vi "Finish.vi"   [LabVIEW 2018]
doc: "This VI is called just before exiting. It is expected to close I/O refnum, save collected data, etc."
uses:
  <vilib>/Rock Robotics/WPI/Utilities/WPI_GetSetVariantRefNum.vi
types:
  T1 = typedef "WPI_JoystickDevRef.ctl" = cluster{"Device":T2}
  T2 = typedef "WPI_JoystickDeviceEnum.ctl" = enum16{"USB 0", "USB 1", "USB 2", "USB 3", "USB 4", "USB 5"}
  T3 = typedef "WPI_SolenoidDevRef.ctl" = cluster{"DevStatus":errorcluster, "Pneumatics Control Module":u8, "Forward Solenoid Channel":T4, "Reverse Solenoid Channel":T4}
  T4 = typedef "WPI_SolenoidChannel.ctl" = enum8{"Solenoid 0", "Solenoid 1", "Solenoid 2", "Solenoid 3", "Solenoid 4", "Solenoid 5", "Solenoid 6", "Solenoid 7", "Invalid"}
  T5 = typedef "WPI_CompressorDevRef.ctl" = cluster{"DevStatus":errorcluster, "Pneumatics Control Module":u8}
  T6 = typedef "WPI_SwitchDevRef.ctl" = cluster{"DevStatus":errorcluster, "DIO Channel":T7, "CntIndex":T8, "Normally Closed":bool}
  T7 = typedef "FPGA_DIOChannel.ctl" = enum8{"DIO 0", "DIO 1", "DIO 2", "DIO 3", "DIO 4", "DIO 5", "DIO 6", "DIO 7", "DIO 8", "DIO 9", "DIO MXP 0", "DIO MXP 1", "DIO MXP 2", "DIO MXP 3", "DIO MXP 4", "DIO MXP 5", "DIO MXP 6", "DIO MXP 7", "DIO MXP 8", "DIO MXP 9", "DIO MXP 10", "DIO MXP 11", "DIO MXP 12", "DIO MXP 13", "DIO MXP 14", "DIO MXP 15", "SPI Port CS1", "SPI Port CS2", "SPI Port CS3", "SPI Port MISO", "SPI Port MOSI", "Invalid"}
  T8 = typedef "FPGA_CounterCtrSystemIndex.ctl" = enum8{"Ctr 0", "Ctr 1", "Ctr 2", "Ctr 3", "Ctr 4", "Ctr 5", "Ctr 6", "Ctr 7", "Invalid"}
  T9 = typedef "WPI_MotorControlDeviceRef.ctl" = cluster{"DeviceStatus":errorcluster, "Type":T10, "PWM":cluster{"PWM Channel":T11, "DeadBand":T12}, "CAN":cluster{"Device Number":u8, "SetOutput VI Ref":variant, "GetOutput VI Ref":variant, "Enable VI Ref":variant, "Disable VI Ref":variant, "Data":variant}, "Invert":bool, "DIO PWM":cluster{"PWM \"Enable\" Channel":T11, "DIOChannel":T7, "PWM Rate":dbl}}
  T10 = typedef "WPI_MotorControlType.ctl" = enum16{"PWM", "CAN", "DIO PWM"}
  T11 = typedef "FPGA_DIOPWMChannel.ctl" = enum8{"PWM 0", "PWM 1", "PWM 2", "PWM 3", "PWM 4", "PWM 5", "PWM 6", "PWM 7", "PWM 8", "PWM 9", "PWM MXP 0", "PWM MXP 1", "PWM MXP 2", "PWM MXP 3", "PWM MXP 4", "PWM MXP 5", "PWM MXP 6", "PWM MXP 7", "PWM MXP 8", "PWM MXP 9", "Invalid"}
  T12 = typedef "WPI_PWMDeadband.ctl" = cluster{"Name":string, "maxPositivePwm":i32, "minPositivePwm":i32, "centerPwm":i32, "maxNegativePwm":i32, "minNegativePwm":i32, "angularRange":u16}
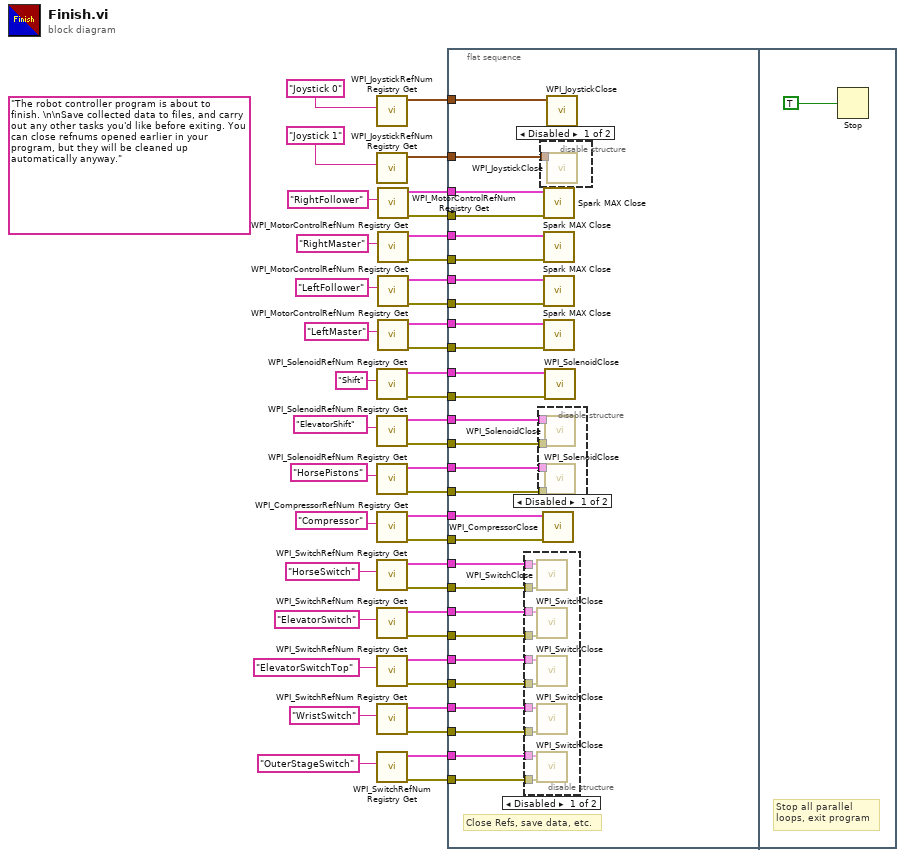
[diagram p0: block diagram]
diagram:
  (unwired) "The robot controller program is about to finish. \n\nSave collected data to files, and carry out any other tasks you'd like before exiting. You can close refnums opened earlier in your program, but they will be cleaned up automatically anyway."
  n1 = call <vilib>:"WPI_JoystickRefNum Registry Get.vi"("refnum name"="Joystick 0") -> ("JoystickDevRef"=w42:T1)  [unwired: 1 in, 9 out]
  n2 = call <vilib>:"WPI_JoystickRefNum Registry Get.vi"("refnum name"="Joystick 1") -> ("JoystickDevRef"=w17:T1)  [unwired: 1 in, 9 out]
  n3 = call <vilib>:"WPI_SolenoidRefNum Registry Get.vi"("refnum name"="Shift") -> ("error out"=w28:errorcluster, "SolenoidDevRef"=w29:T3)  [unwired: 9 in]
  n4 = call <vilib>:"WPI_SolenoidRefNum Registry Get.vi"("refnum name"="ElevatorShift") -> ("error out"=w22:errorcluster, "SolenoidDevRef"=w21:T3)  [unwired: 9 in]
  n5 = call <vilib>:"WPI_SolenoidRefNum Registry Get.vi"("refnum name"="HorsePistons") -> ("error out"=w25:errorcluster, "SolenoidDevRef"=w26:T3)  [unwired: 9 in]
  n6 = call <vilib>:"WPI_CompressorRefNum Registry Get.vi"("refnum name"="Compressor") -> ("error out"=w19:errorcluster, "CompressorDevRef"=w20:T5)  [unwired: 9 in]
  n7 = call <vilib>:"WPI_SwitchRefNum Registry Get.vi"("refnum name"="HorseSwitch") -> ("error out"=w13:errorcluster, "SwitchDevRef"=w14:T6)  [unwired: 9 in]
  n8 = call <vilib>:"WPI_SwitchRefNum Registry Get.vi"("refnum name"="ElevatorSwitch") -> ("error out"=w12:errorcluster, "SwitchDevRef"=w11:T6)  [unwired: 9 in]
  n9 = call <vilib>:"WPI_SwitchRefNum Registry Get.vi"("refnum name"="ElevatorSwitchTop") -> ("error out"=w7:errorcluster, "SwitchDevRef"=w8:T6)  [unwired: 9 in]
  n10 = call <vilib>:"WPI_SwitchRefNum Registry Get.vi"("refnum name"="WristSwitch") -> ("error out"=w6:errorcluster, "SwitchDevRef"=w5:T6)  [unwired: 9 in]
  n11 = call <vilib>:"WPI_SwitchRefNum Registry Get.vi"("refnum name"="OuterStageSwitch") -> ("error out"=w1:errorcluster, "SwitchDevRef"=w2:T6)  [unwired: 9 in]
  n12 = call <vilib>:"WPI_MotorControlRefNum Registry Get.vi"("refnum name"="RightFollower") -> ("error out"=w40:errorcluster, "MotorControlDevRef"=w41:T9)  [unwired: 9 in]
  n13 = call <vilib>:"WPI_MotorControlRefNum Registry Get.vi"("refnum name"="RightMaster") -> ("error out"=w37:errorcluster, "MotorControlDevRef"=w36:T9)  [unwired: 9 in]
  n14 = call <vilib>:"WPI_MotorControlRefNum Registry Get.vi"("refnum name"="LeftFollower") -> ("error out"=w31:errorcluster, "MotorControlDevRef"=w30:T9)  [unwired: 9 in]
  n15 = call <vilib>:"WPI_MotorControlRefNum Registry Get.vi"("refnum name"="LeftMaster") -> ("error out"=w34:errorcluster, "MotorControlDevRef"=w35:T9)  [unwired: 9 in]
  n16 = flat-sequence {
    tunnel: w42 -> [w71]
    tunnel: w41 -> [w70]
    tunnel: w40 -> [w69]
    tunnel: w36 -> [w67]
    tunnel: w37 -> [w68]
    tunnel: w30 -> [w63]
    tunnel: w31 -> [w64]
    tunnel: w35 -> [w66]
    tunnel: w34 -> [w65]
    tunnel: w29 -> [w62]
    tunnel: w28 -> [w61]
    tunnel: w21 -> [w57]
    tunnel: w22 -> [w58]
    tunnel: w26 -> [w60]
    tunnel: w25 -> [w59]
    tunnel: w20 -> [w56]
    tunnel: w19 -> [w55]
    tunnel: w17 -> [w54]
    tunnel: w14 -> [w53]
    tunnel: w13 -> [w52]
    tunnel: w11 -> [w50]
    tunnel: w12 -> [w51]
    tunnel: w8 -> [w49]
    tunnel: w7 -> [w48]
    tunnel: w5 -> [w46]
    tunnel: w6 -> [w47]
    tunnel: w2 -> [w45]
    tunnel: w1 -> [w44]
    frame #0 {
      # "Close Refs, save data, etc."
      n17 = disable-structure shown="Disabled" {
        disable-tunnel: w53 -> [w86 _]
        disable-tunnel: w52 -> [w85 _]
        disable-tunnel: w51 -> [w84 _]
        disable-tunnel: w50 -> [w83 _]
        disable-tunnel: w49 -> [w82 _]
        disable-tunnel: w48 -> [w81 _]
        disable-tunnel: w47 -> [w80 _]
        disable-tunnel: w46 -> [w79 _]
        disable-tunnel: w45 -> [w78 _]
        disable-tunnel: w44 -> [w77 _]
        frame Disabled {
          n18 = call <vilib>:"WPI_SwitchClose.vi"("error in (no error)"=w85, "SwitchDevRef"=w86) -> ()  [unwired: 9 in, 1 out]
          n19 = call <vilib>:"WPI_SwitchClose.vi"("error in (no error)"=w84, "SwitchDevRef"=w83) -> ()  [unwired: 9 in, 1 out]
          n20 = call <vilib>:"WPI_SwitchClose.vi"("error in (no error)"=w81, "SwitchDevRef"=w82) -> ()  [unwired: 9 in, 1 out]
          n21 = call <vilib>:"WPI_SwitchClose.vi"("error in (no error)"=w80, "SwitchDevRef"=w79) -> ()  [unwired: 9 in, 1 out]
          n22 = call <vilib>:"WPI_SwitchClose.vi"("error in (no error)"=w77, "SwitchDevRef"=w78) -> ()  [unwired: 9 in, 1 out]
        }
        frame Enabled {
        }
      }
      n23 = disable-structure shown="Disabled" {
        disable-tunnel: w60 -> [w75 _]
        disable-tunnel: w59 -> [w74 _]
        disable-tunnel: w58 -> [w73 _]
        disable-tunnel: w57 -> [w72 _]
        frame Disabled {
          n24 = call <vilib>:"WPI_SolenoidClose.vi"("error in (no error)"=w73, "SolenoidDevRef"=w72) -> ()  [unwired: 9 in, 1 out]
          n25 = call <vilib>:"WPI_SolenoidClose.vi"("error in (no error)"=w74, "SolenoidDevRef"=w75) -> ()  [unwired: 9 in, 1 out]
        }
        frame Enabled {
        }
      }
      n26 = disable-structure shown="Disabled" {
        disable-tunnel: w54 -> [w76 _]
        frame Disabled {
          n27 = call <vilib>:"WPI_JoystickClose.vi"("JoystickDevRef"=w76) -> ()  [unwired: 11 out]
        }
        frame Enabled {
        }
      }
      n28 = call <vilib>:"WPI_CompressorClose.vi"("error in (no error)"=w55, "CompressorDevRef"=w56) -> ()  [unwired: 9 in, 1 out]
      n29 = call <vilib>:"Spark MAX Close.vi"("error in"=w69, "MotorControlDeviceRef"=w70) -> ()  [unwired: 9 in, 1 out]
      n30 = call <vilib>:"Spark MAX Close.vi"("error in"=w68, "MotorControlDeviceRef"=w67) -> ()  [unwired: 9 in, 1 out]
      n31 = call <vilib>:"Spark MAX Close.vi"("error in"=w64, "MotorControlDeviceRef"=w63) -> ()  [unwired: 9 in, 1 out]
      n32 = call <vilib>:"Spark MAX Close.vi"("error in"=w65, "MotorControlDeviceRef"=w66) -> ()  [unwired: 9 in, 1 out]
      n33 = call <vilib>:"WPI_SolenoidClose.vi"("error in (no error)"=w61, "SolenoidDevRef"=w62) -> ()  [unwired: 9 in, 1 out]
      n34 = call <vilib>:"WPI_JoystickClose.vi"("JoystickDevRef"=w71) -> ()  [unwired: 11 out]
    }
    frame #1 {
      # "Stop all parallel\nloops, exit program"
      n35 = Stop(stop? (T)=TRUE ("Quit")) -> ()
    }
  }
